vi "svx_Polar_Draw_Angle_Label.vi"(5 "[user-specified font]":T3, 6 "text color(black)":u32(colorbox), 7 "desired font(Application)":T2(ring)=enum."Application Font", 8 "grid measurements":T1={"pixel center"={"x"=175, "y"=175}, "scale factors"={"a"=7195.980240002514, "b"=0.0, "log?"=FALSE}, "grid color"=3381657, "start angle"=0.0, "end angle"=360.0, "tick length"=159, "pixel radius"=157} {"end angle" format="%.2f"; "start angle" format="%.2f"; "scale factors"."b" format="%.2f"; "scale factors"."a" format="%.2f"}, 9 "shaft rotating direction":u16(ring) items=["CCW", "CW"], 10 "probe position":u16, 11 "Picture":picture) -> (3 "new picture":picture)   [LabVIEW 2017, in "SVX Polar Plot.xctl"]
uses:
  <vilib>/addons/_XControls/Polar Plot/SVX Polar Plot.xctl
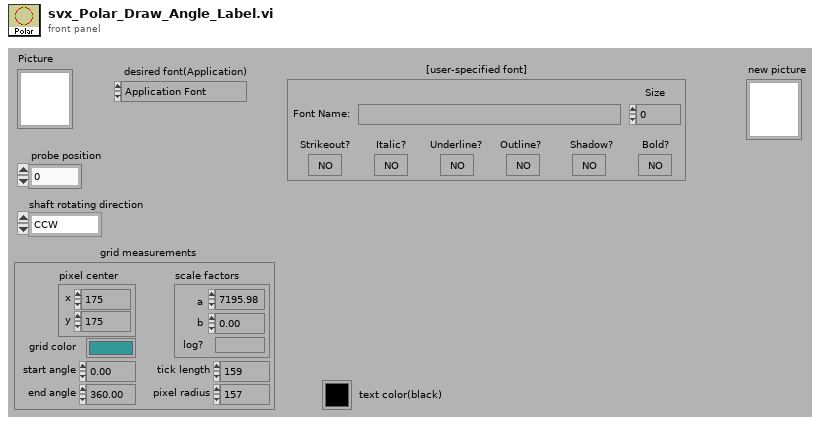
[diagram p1: front panel]
types:
  T1 = cluster{"pixel center":cluster{"x":i16, "y":i16}, "scale factors":cluster{"a":dbl, "b":dbl, "log?":bool}, "grid color":u32, "start angle":dbl, "end angle":dbl, "tick length":i16, "pixel radius":i32}
  T2 = enum16{"User-specified Font", "Application Font", "System Font", "Dialog Font"}
  T3 = cluster{"Font Name:":string, "Size":i16, "Strikeout?":bool, "Italic?":bool, "Underline?":bool, "Outline?":bool, "Shadow?":bool, "Bold?":bool}
  T4 = cluster{"horizontal":enum16{"left", "center", "right"}, "vertical":enum16{"top", "center", "bottom"}}[]
  T5 = cluster{"horizontal":enum16{"left", "center", "right"}, "vertical":enum16{"top", "center", "bottom"}}
  T6 = enum16{"None", "Stacked", "Clockwise", "Counterclockwise"}
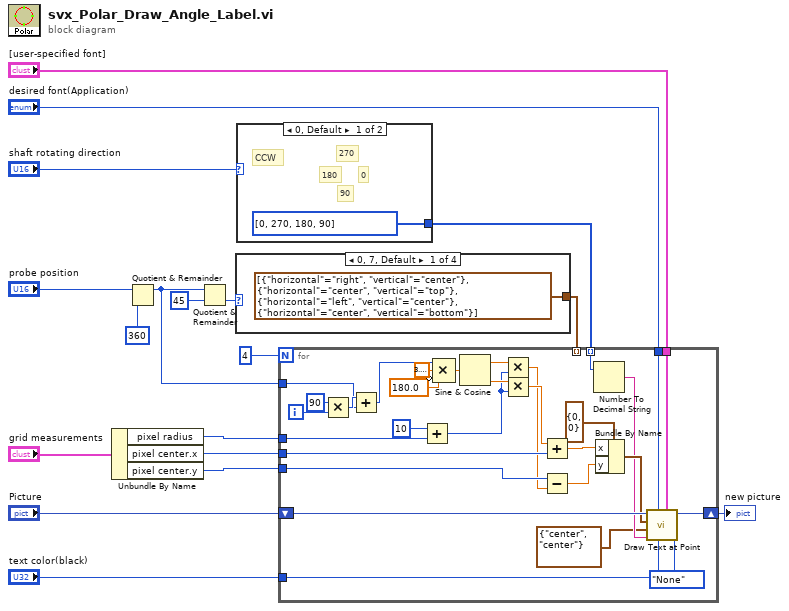
[diagram p0: block diagram]
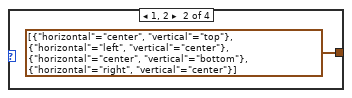
[diagram p2: hidden frame]
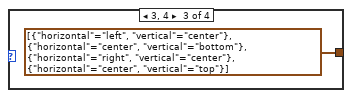
[diagram p3: hidden frame]
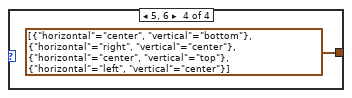
[diagram p4: hidden frame]
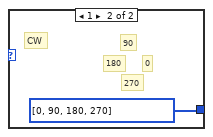
[diagram p5: hidden frame]
diagram:
  n1 = Unbundle By Name("grid measurements") -> ("pixel radius"=w11:i32, "pixel center.x"=w10:i16, "pixel center.y"=w9:i16)
  n2 = Quotient & Remainder(x="probe position", y=u16 360) -> (x-y*floor(x/y)=w12:u16)  [unwired: 1 out]
  n3 = Quotient & Remainder(x=w12, y=u16 45) -> (floor(x/y)=w16:u16)  [unwired: 1 out]
  n4 = case shown="0, 7, Default" w16 {
    tunnel: [T4 [{"horizontal"=enum."right", "vertical"=enum."center"}, {"horizontal"=enum."center", "vertical"=enum."top"}, {"horizontal"=enum."left", "vertical"=enum."center"}, {"horizontal"=enum."center", "vertical"=enum."bottom"}] T4 [{"horizontal"=enum."center", "vertical"=enum."top"}, {"horizontal"=enum."left", "vertical"=enum."center"}, {"horizontal"=enum."center", "vertical"=enum."bottom"}, {"horizontal"=enum."right", "vertical"=enum."center"}] T4 [{"horizontal"=enum."left", "vertical"=enum."center"}, {"horizontal"=enum."center", "vertical"=enum."bottom"}, {"horizontal"=enum."right", "vertical"=enum."center"}, {"horizontal"=enum."center", "vertical"=enum."top"}] T4 [{"horizontal"=enum."center", "vertical"=enum."bottom"}, {"horizontal"=enum."right", "vertical"=enum."center"}, {"horizontal"=enum."center", "vertical"=enum."top"}, {"horizontal"=enum."left", "vertical"=enum."center"}]] -> w8
    frame 0, 7, Default {
    }
    frame 1, 2 {
    }
    frame 3, 4 {
    }
    frame 5, 6 {
    }
  }
  n5 = case shown="0, Default" "shaft rotating direction" {
    tunnel: [i32[] [0, 270, 180, 90] i32[] [0, 90, 180, 270]] -> w6
    frame 0, Default {
      # "180"
      # "90"
      # "0"
      # "270"
      # "CCW"
    }
    frame 1 {
      # "180"
      # "270"
      # "0"
      # "90"
      # "CW"
    }
  }
  n6 = for {
    N: 4 -> [_]
    tunnel: w12 -> [w51]
    tunnel: w11 -> [w29]
    tunnel: w10 -> [w44]
    tunnel: w9 -> [w32]
    tunnel: w8 -> [_] mode=indexing
    tunnel: w6 -> [w43] mode=indexing
    tunnel: "desired font(Application)" -> [w37]
    tunnel: "[user-specified font]" -> [w38]
    shift-right: [w39] -> w3
    shift-left: "Picture" -> [w40]
    tunnel: "text color(black)" -> [w30]
    i -> [w54]
    n7 = Multiply(x=90, y=w54) -> (x*y=w52:i32)
    n8 = Add(x=w52, y=w51) -> (x+y=w45:i32)
    n9 = Add(x=10, y=w29) -> (x+y=w27:i32)
    n10 = Compound Arithmetic op=MULTIPLY(w45, 3.141592653589793, invert 180.0 ("value")) -> (w48:dbl)
    n11 = Sine & Cosine(0:w48) -> (1:w49:dbl, 2:w50:dbl)
    n12 = Multiply(x=w49, y=w27) -> (x*y=w31:dbl)
    n13 = Multiply(x=w50, y=w27) -> (x*y=w33:dbl)
    n14 = Add(x=w33, y=w44) -> (x+y=w42:dbl)
    n15 = Subtract(x=w32, y=w31) -> (x-y=w41:dbl)
    n16 = Number To Decimal String(number=w43) -> (decimal integer string=w35:string)  [unwired: 1 in]
    n17 = Bundle By Name(cluster=cluster{"x":i16, "y":i16} {"x"=0, "y"=0} ("origin"), "x"=w42, "y"=w41) -> (w36:cluster{"x":i16, "y":i16})
    n18 = call <vilib>:"Draw Text at Point.vi"("text orientation"=T6."None", "[user-specified font]"=w38, "text color(black)"=w30, "desired font(Application)"=w37, "text"=w35, "alignment(left, top)"=T5 {"horizontal"=enum."center", "vertical"=enum."center"}, "origin"=w36, "picture"=w40) -> ("new picture"=w39:picture)  [unwired: 2 in, 1 out]
  }
  "new picture" <- w3
